vi "日志信息主动发送(子VI).vi"   [LabVIEW 2016, in "数据传输系统.lvlib"]
types:
  T1 = typedef "LVDateTimeRec.ctl" = cluster{"秒数的小数部分":dbl, "秒":i32, "分":i32, "时":i32, "日":i32, "月":i32, "年":i32, "天数（周）":i32, "天数（年）":i32, "DST":i32}
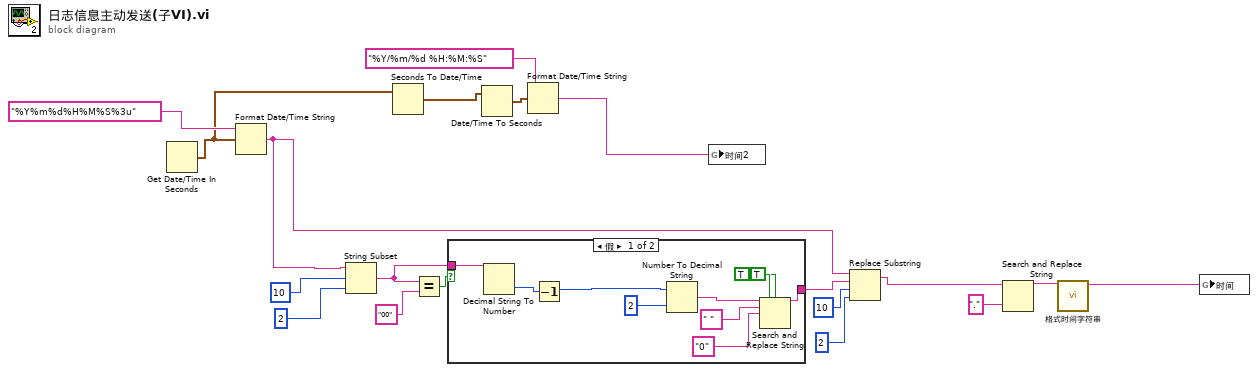
[diagram p0: block diagram]
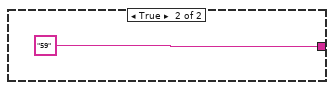
[diagram p2: hidden frame]
diagram:
  n1 = Get Date/Time In Seconds() -> (seconds since 1Jan1904=w4:timestamp)
  n2 = Format Date/Time String(time format string (%c)="%Y%m%d%H%M%S%3u" ("时间格式字符串(%c)"), seconds (now)=w4) -> (date/time string=w8:string)  [unwired: 1 in]
  n3 = String Subset(string=w8, offset (0)=10 ("偏移量(0)"), length (rest)=2 ("长度（子字符串长度）")) -> (substring=w16:string)
  n4 = Seconds To Date/Time(time stamp (now)=w4) -> (date time rec=w5:T1)  [unwired: 1 in]
  n5 = Equal?(x=w16, y="00") -> (x = y?=w15:bool)
  n6 = case shown="假" w15 {
    tunnel: w16 -> [w29 _]
    tunnel: [w21 "59" ("y")] -> w17
    frame False {
      n7 = Decimal String To Number(string=w29) -> (number=w28:i32)  [unwired: 2 in, 1 out]
      n8 = Decrement(x=w28) -> (x-1=w22:i32)
      n9 = Number To Decimal String(number=w22, width (-)=i16 2 ("宽度(-)")) -> (decimal integer string=w24:string)
      n10 = Search and Replace String(replace all?=TRUE ("替换全部？(F)"), case sensitive?=TRUE ("忽略大小写？(F)"), input string=w24, search string=" " ("搜索字符串"), replace string="0" ("替换字符串(\"\")")) -> (result string=w21:string)  [unwired: 3 in, 3 out]
    }
    frame True {
    }
  }
  n11 = Date/Time To Seconds(2:w5) -> (0:w7:timestamp)  [unwired: 1 in]
  n12 = Format Date/Time String(time format string (%c)="%Y/%m/%d %H:%M:%S" ("时间格式字符串(%c)"), seconds (now)=w7) -> (date/time string=w3:string)  [unwired: 1 in]
  n13 = global write "全局 时间2.vi" "时间2"(w3) -> ()
  n14 = Replace Substring(2:2 ("长度（子字符串长度）"), 3:10 ("偏移量(0)"), 4:w17, 5:w8) -> (1:w9:string)  [unwired: 1 out]
  n15 = Search and Replace String(input string=w9, search string="." ("搜索字符串")) -> (result string=w1:string)  [unwired: 6 in, 3 out]
  n16 = call "格式时间字符串.vi"("字符串"=w1) -> ("连接的字符串"=w10:string)  [unwired: 10 in]
  n17 = global write "全局 水样时间.vi" "时间"(w10) -> ()
